vi "TEST_Alpha.vi"() -> ()   [LabVIEW 2021, in "Picture2D.lvlib"]
uses:
  Picture2D/Picture2D.lvlib
  Picture/Image.lvclass
  C:/GitHub/danyallard/Picture2D/src/IDrawable/IDrawable.lvclass
  Collection/Collection.lvclass
  PointSpecialized/PointSpecialized.lvclass
  C:/GitHub/danyallard/Picture2D/src/Point/Point.lvclass
  ColorRGBA/ColorRGBA.lvclass
  C:/GitHub/danyallard/Picture2D/src/Color/Color.lvclass
  ColorRGB/ColorRGB.lvclass
  PointSpecialized/PointSpecialized.lvclass/PointSpecialized.ctl
  <vilib>/picture/picture.llb/imagedata.ctl
panel:
  out "2D Picture 4":picture
  in  "X":i16(slide) scale=-50.0..250.0
  in  "Y":i16(slide) scale=250.0..-50.0
  in  "Alpha (255 opaque) CLA":u8(slide)=255 scale=0.0..255.0
  out "2D Picture 3":picture
  in  "Alpha (255 opaque) Heart":u8(slide)=255 scale=0.0..255.0
  out "2D Picture 2":picture
  out "image data 2":T1
  out "x*y 2":i32
  out "x*y":i32
  out "size(s)":i32
  out "24-bit pixmap":u32[][](array[colorbox])
  out "image data":T1
  out "2D Picture":picture
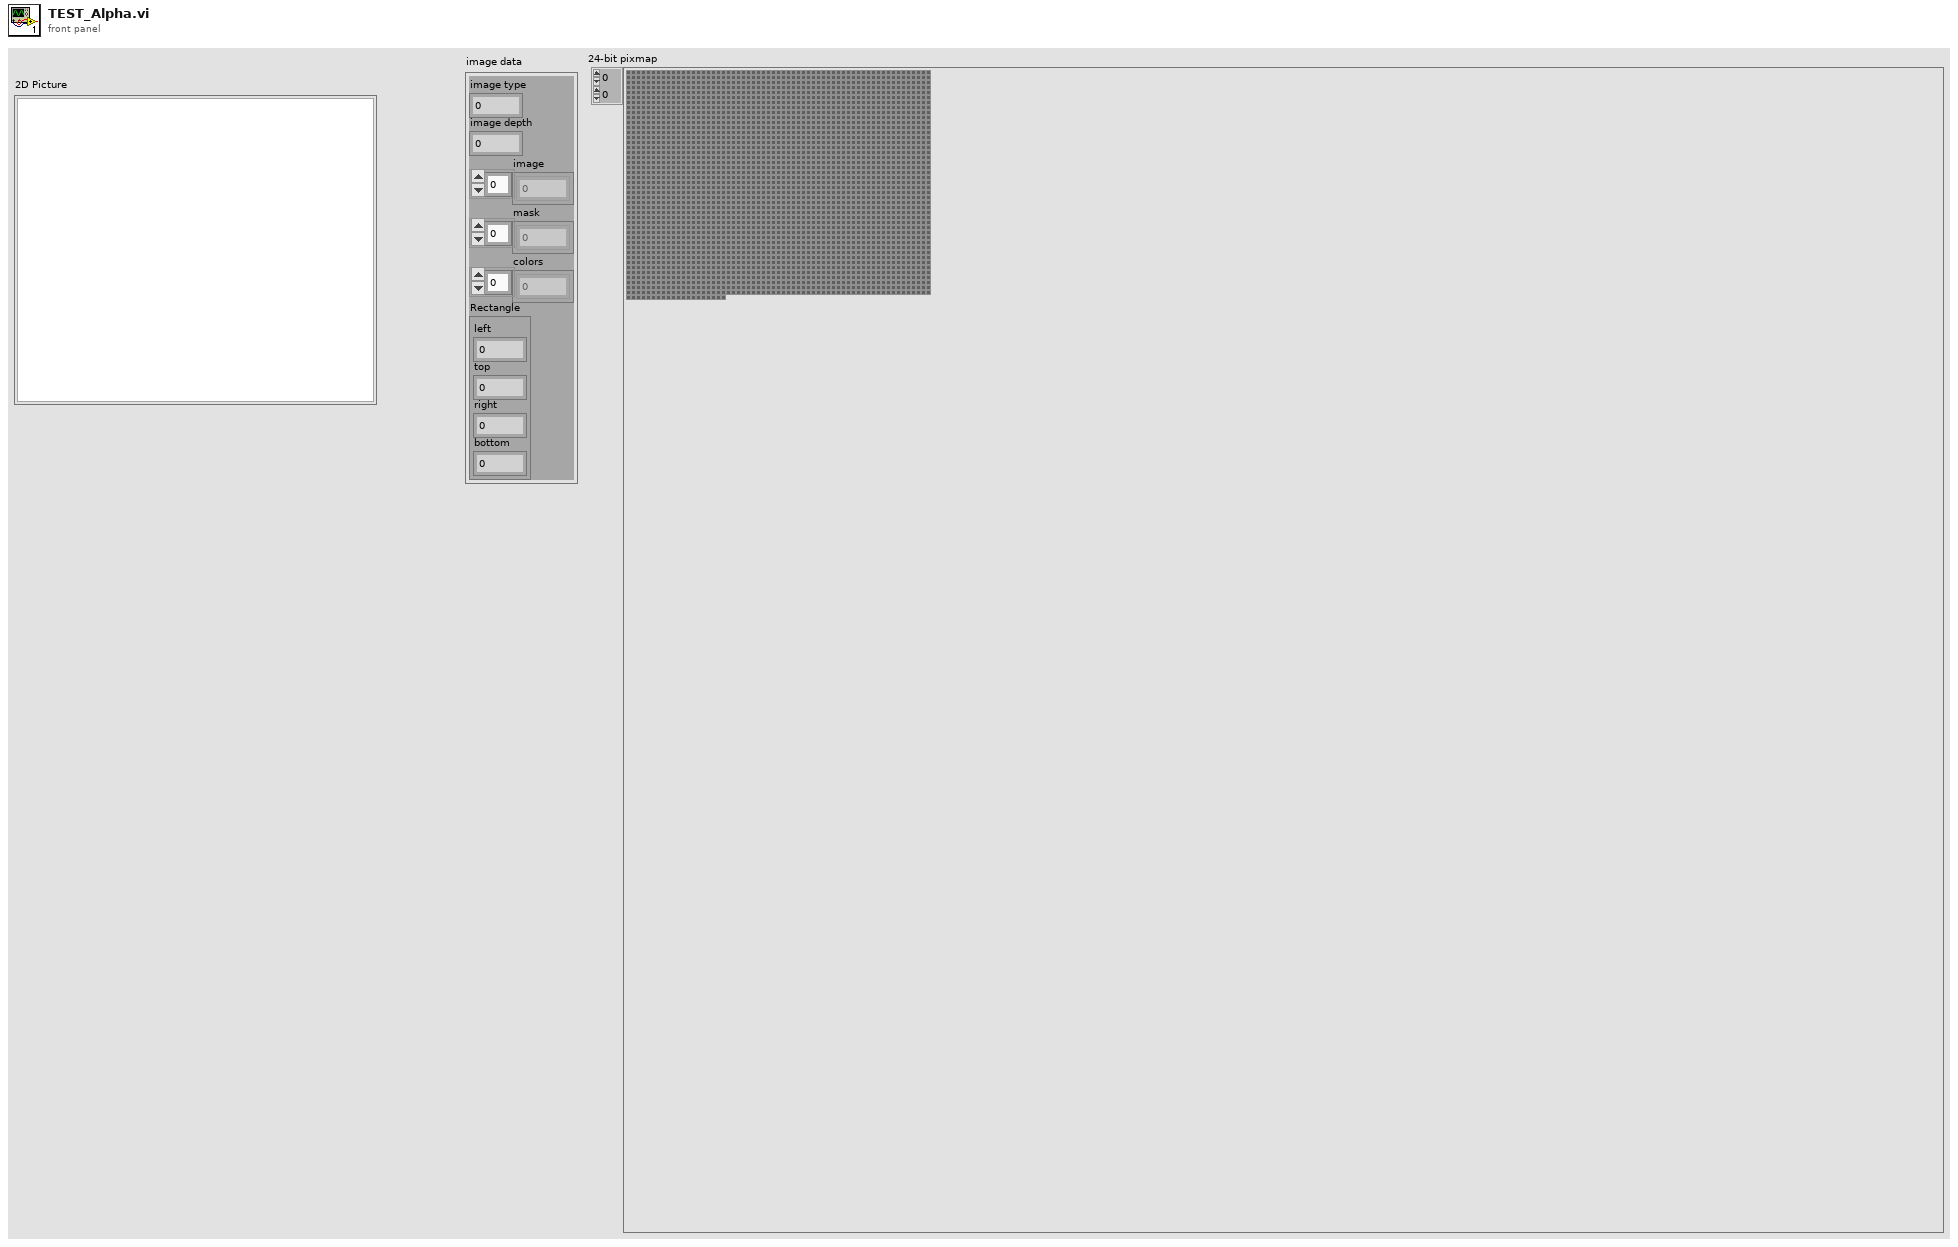
[diagram p1: front panel]
types:
  T1 = typedef "imagedata.ctl" = cluster{"image type":i32, "image depth":i32, "image":u8[], "mask":u8[], "colors":u32[], "Rectangle":cluster{"left":i16, "top":i16, "right":i16, "bottom":i16}}
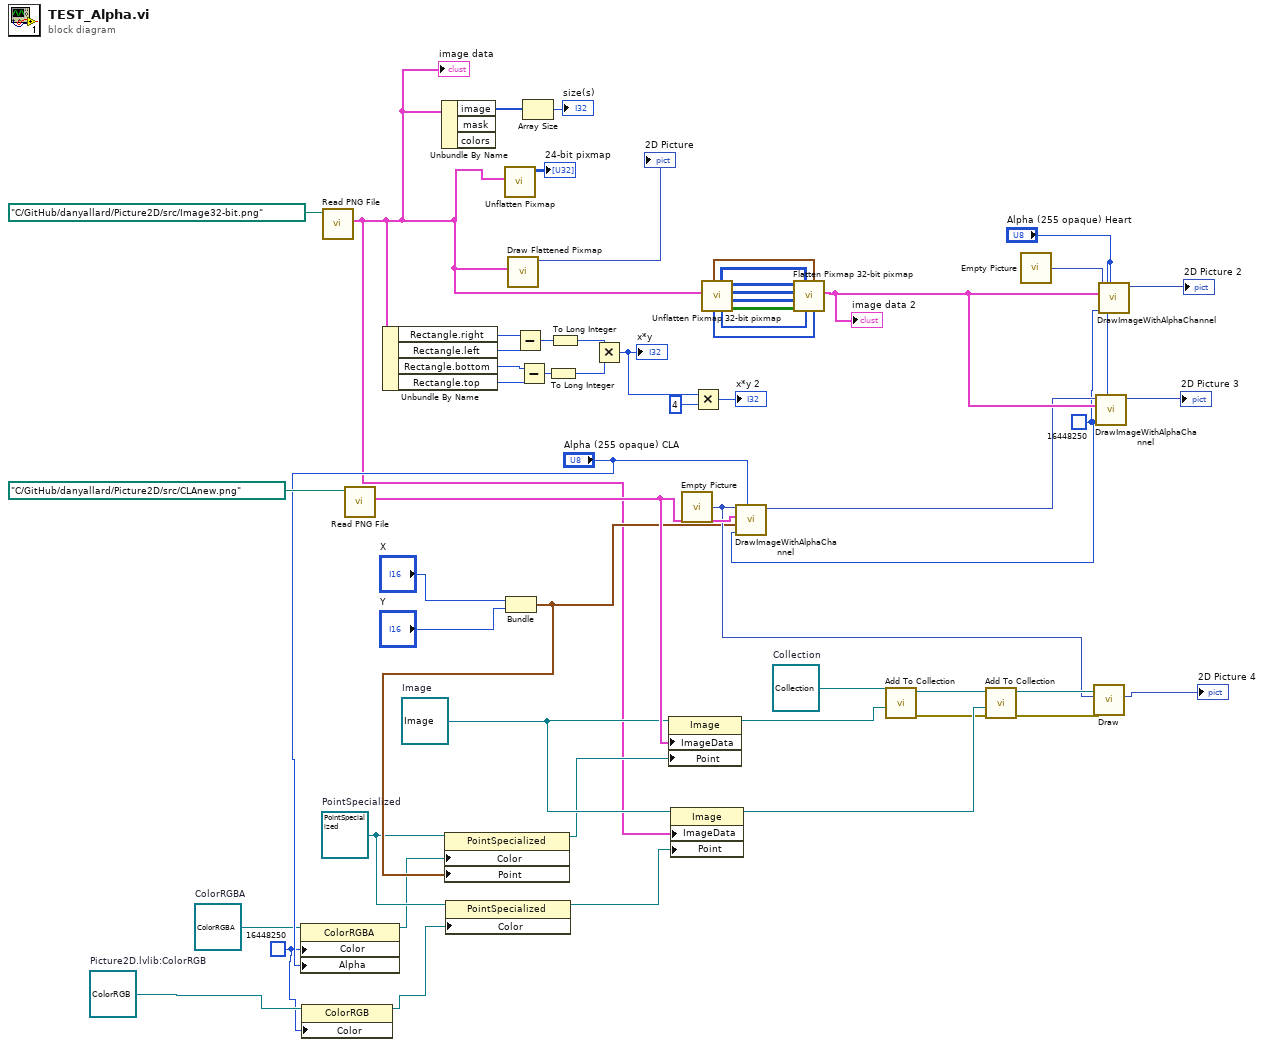
[diagram p0: block diagram]
diagram:
  w4 = refnum<class "ColorRGB.lvclass"> refnum  # Picture2D.lvlib:ColorRGB
  w2 = u32 16448250 ("Color")
  w7 = refnum<class "ColorRGBA.lvclass"> refnum  # ColorRGBA
  w11 = refnum<class "PointSpecialized.lvclass"> refnum  # PointSpecialized
  w20 = refnum<class "Collection.lvclass"> refnum  # Collection
  w21 = refnum<class "Image.lvclass"> refnum  # Image
  w23 = u32 16448250 ("Background Color")
  n1 = property class="ColorRGBA"(reference=w7, "Color"=w2, "Alpha"="Alpha (255 opaque) CLA") -> (reference out=w9:refnum<class "ColorRGBA.lvclass">)  [unwired: 1 in, 1 out]
  n2 = property class="ColorRGB"(reference=w4, "Color"=w2) -> (reference out=w3:refnum<class "ColorRGB.lvclass">)  [unwired: 1 in, 1 out]
  n3 = call <vilib>:"Read PNG File.vi"("path to PNG file"=path "C:/GitHub/danyallard/Picture2D/src/Image32-bit.png") -> ("image data"=w1:T1)  [unwired: 8 in, 2 out]
  "image data" <- w1
  n4 = call <vilib>:"Read PNG File.vi"("path to PNG file"=path "C:/GitHub/danyallard/Picture2D/src/CLAnew.png") -> ("image data"=w22:T1)  [unwired: 8 in, 2 out]
  n5 = Unbundle By Name(w1) -> ("Rectangle.right"=w51:i16, "Rectangle.left"=w50:i16, "Rectangle.bottom"=w49:i16, "Rectangle.top"=w48:i16)
  n6 = Unbundle By Name(w1) -> ("image"=w53:u8[])  [unwired: 2 out]
  n7 = property class="PointSpecialized"(reference=w11, "Color"=w3) -> (reference out=w10:refnum<class "PointSpecialized.lvclass">)  [unwired: 1 in, 1 out]
  n8 = call <vilib>:"Unflatten Pixmap.vi"("image data"=w1) -> ("24-bit pixmap"=→"24-bit pixmap":u32[][])  [unwired: 4 in, 6 out]
  n9 = Bundle("X"="X", "Y"="Y") -> (w13:cluster{"X":i16, "Y":i16})  [unwired: 1 in]
  n10 = property class="PointSpecialized"(reference=w11, "Color"=w9, "Point"=w13) -> (reference out=w12:refnum<class "PointSpecialized.lvclass">)  [unwired: 1 in, 1 out]
  n11 = call <vilib>:"Draw Flattened Pixmap.vi"("image data"=w1) -> ("new picture"=→"2D Picture":picture)  [unwired: 8 in]
  n12 = Subtract(x=w51, y=w50) -> (x-y=w47:i16)
  n13 = Subtract(x=w49, y=w48) -> (x-y=w46:i16)
  n14 = Array Size(array=w53) -> (size(s)=→"size(s)":i32)
  n15 = To Long Integer(number=w46) -> (32bit integer=w44:i32)
  n16 = To Long Integer(number=w47) -> (32bit integer=w45:i32)
  n17 = Multiply(x=w45, y=w44) -> (x*y=w43:i32)
  "x*y" <- w43
  n18 = property class="Image"(reference=w21, "ImageData"=w22, "Point"=w12) -> (reference out=w19:refnum<class "Image.lvclass">)  [unwired: 1 in, 1 out]
  n19 = property class="Image"(reference=w21, "ImageData"=w1, "Point"=w10) -> (reference out=w18:refnum<class "Image.lvclass">)  [unwired: 1 in, 1 out]
  n20 = call "Empty Picture"() -> ("empty picture"=w14:picture)
  n21 = Multiply(x=w43, y=4) -> (x*y=→"x*y 2":i32)
  n22 = call "Unflatten Pixmap 32-bit pixmap.vi"("image data"=w1) -> ("1-bit pixmap"=w37:bool[][], "4-bit pixmap"=w38:u8[][], "8-bit pixmap"=w39:u8[][], "24-bit pixmap"=w40:u32[][], "colors"=w36:u32[], "32-bit pixmap"=w34:u32[][], "mask"=w35:u8[], "top left"=w33:cluster{"x":i16, "y":i16})  [unwired: 3 in]
  n23 = call "DrawImageWithAlphaChannel.vi"("Alpha (255 opaque)"="Alpha (255 opaque) CLA", "Background Color"=w23, "Insertion Point(x,y)"=w13, "image data"=w22, "2D Picture in"=w14) -> ("2D Picture out"=w27:picture)  [unwired: 6 in]
  n24 = call "Flatten Pixmap 32-bit pixmap.vi"("mask"=w35, "top left"=w33, "colors"=w36, "32-bit pixmap"=w34, "1-bit pixmap"=w37, "4-bit pixmap"=w38, "8-bit pixmap"=w39, "24-bit pixmap"=w40) -> ("image data"=w28:T1)  [unwired: 3 in]
  "image data 2" <- w28
  n25 = call-dynamic "Add To Collection.vi"("IDrawable"=w19, "Collection in"=w20) -> ("error out"=w6:errorcluster, "Collection out"=w17:refnum<class "Collection.lvclass">)  [unwired: 8 in]
  n26 = call-dynamic "Add To Collection.vi"("error in (no error)"=w6, "IDrawable"=w18, "Collection in"=w17) -> ("error out"=w5:errorcluster, "Collection out"=w16:refnum<class "Collection.lvclass">)  [unwired: 7 in]
  n27 = call "Empty Picture"() -> ("empty picture"=w31:picture)
  n28 = call-dynamic "Draw.vi"("error in (no error)"=w5, "2D Picture in"=w14, "Collection in"=w16) -> ("2D Picture out"=→"2D Picture 4":picture)  [unwired: 6 in, 2 out]
  n29 = call "DrawImageWithAlphaChannel.vi"("Alpha (255 opaque)"="Alpha (255 opaque) Heart", "Background Color"=w23, "image data"=w28, "2D Picture in"=w27) -> ("2D Picture out"=→"2D Picture 3":picture)  [unwired: 7 in]
  n30 = call "DrawImageWithAlphaChannel.vi"("Alpha (255 opaque)"="Alpha (255 opaque) Heart", "Background Color"=w23, "image data"=w28, "2D Picture in"=w31) -> ("2D Picture out"=→"2D Picture 2":picture)  [unwired: 7 in]
